vi "Decide Loop.vi"   [LabVIEW 2009]
uses:
  <vilib>/Platform/TimedLoop/XDataNode/XDataNode.xnode
  <vilib>/Platform/TimedLoop/XDataNode/nitl_modes.ctl
  <vilib>/Platform/TimedLoop/XDataNode/XDNodeRunTimeDep.lvlib
  <vilib>/Platform/TimedLoop/XDataNode/wakeup.ctl
  <vilib>/Platform/TimedLoop/XDataNode/timing_clust.ctl
  <vilib>/Platform/TimedLoop/XDataNode/loadlvalarms.vi
types:
  T1 = typedef "XDNodeRunTimeDep.lvlib/timing_clust.ctl" = cluster{"Expected End [f-1]":u64, "Actual End [f-1]":u64, "Finished Late? [f-1]":bool, "Expected End [i-1]":u64, "Actual End [i-1]":u64, "Finished Late? [i-1]":bool, "Expected Start [i]":u64, "Actual Start [i]":u64, "Expected Start [f]":u64, "Actual Start [f]":u64, "Source Name":string, "Structure Name":string, "Period":i64, "Deadline":i64, "Offset":i64, "Start":i64, "Priority":i32, "Timeout":i32, "Mode":T2, "Wakeup Reason":T3, "Error":errorcluster, "Source Type":string, "Secondary Source Type":string, "Global End Time":u64, "Global Start Time":u64, "Frame Duration":u64, "Iteration Duration":u64, "Assigned CPU":i32, "I/O Scan Engine Mode":u32}
  T2 = typedef "XDNodeRunTimeDep.lvlib/nitl_modes.ctl" = enum32{"No Change", "Process missed periods, maintain original phase", "Discard missed periods, maintain original phase", "Process missed periods, ignore original phase", "Discard missed periods, ignore original phase"}
  T3 = typedef "XDNodeRunTimeDep.lvlib/wakeup.ctl" = enum32{"Normal", "Aborted", "Asynchronous wakeup", "Timing source error", "Timed loop error", "Timeout"}
  T4 = typedef "GPS Data.ctl" = cluster{"Latitude":dbl, "Longitude":dbl}
  T5 = typedef "SICK Array.ctl" = u16[]
  T6 = typedef "Motor Command.ctl" = cluster{"Speed":i16, "Turn":i16}
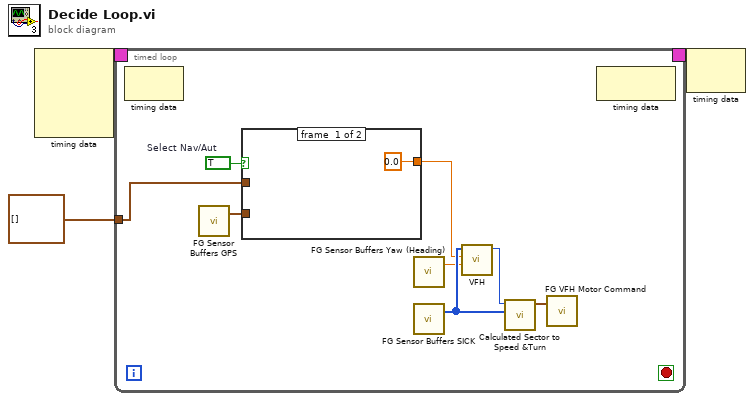
[diagram p0: block diagram]
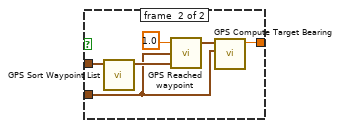
[diagram p2: hidden frame]
diagram:
  n1 = node-c288() -> (w3:T1)  [unwired: 4 in]
  n2 = timed-loop {
    timing: w3 -> [_]
    timing-out: [_] -> w2
    tunnel: cluster{"Longitude":dbl, "Latitude":dbl}[] [] ("Unsorted Waypoints") -> [w11]
    stop <- _ stop-if-true
    w8 = TRUE  # Select Nav/Aut
    n3 = node-c288() -> ()  [unwired: 1 in, 1 out]
    n4 = call "FG Sensor Buffers GPS.vi"() -> ("GPS Buffer out"=w9:T4)  [unwired: 3 in]
    n5 = case shown="True" w8 {
      tunnel: w11 -> [_ w18]
      tunnel: w9 -> [_ w14]
      tunnel: [0.0 ("Target Bearing (degrees)") w13] -> w5
      frame #0 {
      }
      frame #1 {
        n6 = call "GPS Sort Waypoint List.vi"("Unsorted Waypoint List"=w18) -> ("Sorted Waypoints"=w17:T4[])  [unwired: 10 in]
        n7 = call "GPS Reached waypoint.vi"("Sorted GPS Waypoint List In (Lat/Long)"=w17, "Current co-ordinates"=w14, "Required distance to target (meters)"=1.0) -> ("GPS Waypoint List Out (Lat/Long)"=w15:cluster{"Latitude":dbl, "Longitude":dbl}[])  [unwired: 2 in]
        n8 = call "GPS Compute Target Bearing.vi"("Current co-ordinates"=w14, "GPS Waypoint List Out"=w15) -> ("Target Bearing (degrees)"=w13:dbl)  [unwired: 8 in]
      }
    }
    n9 = call "FG Sensor Buffers Yaw (Heading).vi"() -> ("Yaw Buffer Out"=w4:dbl)  [unwired: 3 in]
    n10 = call "FG Sensor Buffers SICK.vi"() -> ("SICK Buffer out"=w6:T5)  [unwired: 3 in]
    n11 = call "VFH.vi"("Compass Bearing (degrees)"=w4, "Target Bearing (degrees)"=w5, "RAW SICK Data"=w6) -> ("Calculated sector"=w7:i16)  [unwired: 8 in]
    n12 = call "Calculated Sector to Speed &Turn.vi"("RAW SICK Data"=w6, "Calculated Sector"=w7) -> ("Motor Commands"=w10:T6)  [unwired: 9 in]
    n13 = call "FG VFH Motor Command.vi"("Motor Command in"=w10) -> ()  [unwired: 2 in, 1 out]
    n14 = node-c288() -> ()  [unwired: 1 in, 1 out]
  }
  n15 = node-c288(w2) -> ()  [unwired: 1 out]
